vi "I2C Read Byte.vi"(8 "error in (no error)":errorcluster, 10 "Ack? (F:False)":bool, 11 "I2C Task In":T1) -> (0 "error out":errorcluster, 2 "Data Byte":u8 format="%x", 3 "I2C Task Out":T1)   [LabVIEW 2017, in "I2C.lvlib"]
doc: "Reads a single byte from a slave device on the I2C port."
uses:
  <vilib>/robotics/Protocols/I2C/DAQmx/I2C.lvlib
  <vilib>/robotics/Protocols/I2C/DAQmx/Private/I2C Tasks.ctl
  <vilib>/DAQmx/read.llb/DAQmx Read (Digital Bool 1Line 1Point).vi
  <vilib>/DAQmx/miscellaneous.llb/DAQmx Fill In Error Info.vi
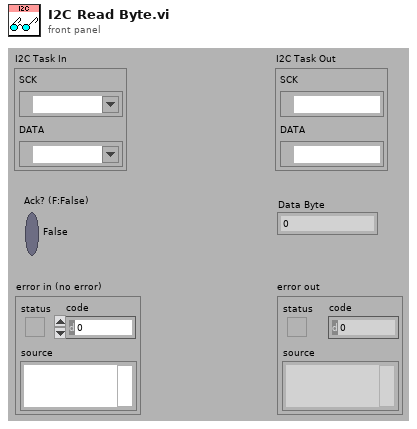
[diagram p1: front panel]
types:
  T1 = typedef "I2C.lvlib/I2C Tasks.ctl" = cluster{"SCK":refnum<k21>, "DATA":refnum<k21>}
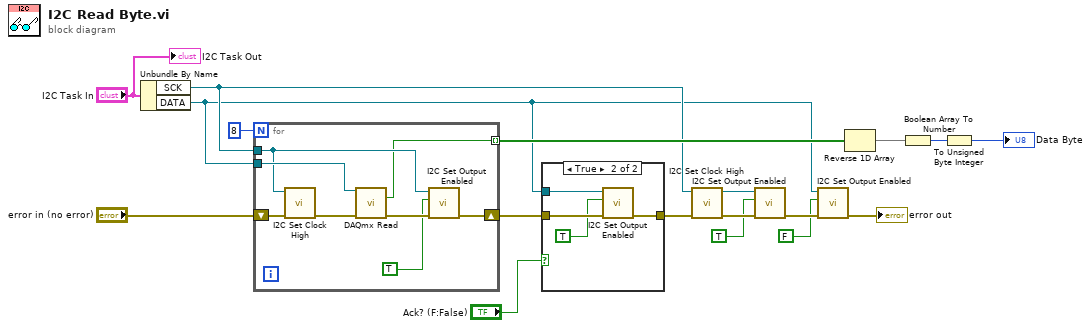
[diagram p0: block diagram]
diagram:
  n1 = Unbundle By Name("I2C Task In") -> ("SCK"=w9:refnum<k21>, "DATA"=w5:refnum<k21>)
  n2 = for {
    N: 8 -> [_]
    shift-right: [w19] -> w11
    shift-left: "error in (no error)" -> [w26]
    tunnel: [w20] -> w14 mode=indexing
    tunnel: w9 -> [w23]
    tunnel: w5 -> [w25]
    n3 = call <vilib>:"I2C Set Clock High.vi"("error in (no error)"=w26, "Task In"=w23) -> ("error out"=w24:errorcluster)  [unwired: 8 in, 1 out]
    n4 = call-poly <vilib>:"DAQmx Read.vi"("task/channels in"=w25, "error in"=w24) -> ("data"=w20:bool, "error out"=w22:errorcluster)  [unwired: 11 in, 1 out]
    n5 = call <vilib>:"I2C Set Output Enabled.vi"("error in (no error)"=w22, "Output Enabled (T:Enable)"=TRUE, "Task In"=w23) -> ("error out"=w19:errorcluster)  [unwired: 7 in, 1 out]
  }
  n6 = case shown="True" "Ack? (F:False)" {
    tunnel: w5 -> [_ w31]
    tunnel: w11 -> [w27 w30]
    tunnel: [w27 w28] -> w10
    frame False {
    }
    frame True {
      n7 = call <vilib>:"I2C Set Output Enabled.vi"("error in (no error)"=w30, "Output Enabled (T:Enable)"=TRUE ("DO.Tristate"), "Task In"=w31) -> ("error out"=w28:errorcluster)  [unwired: 7 in, 1 out]
    }
  }
  n8 = call <vilib>:"I2C Set Clock High.vi"("error in (no error)"=w10, "Task In"=w9) -> ("error out"=w7:errorcluster, "Task Out"=w8:refnum<k21>)  [unwired: 8 in]
  n9 = call <vilib>:"I2C Set Output Enabled.vi"("error in (no error)"=w7, "Output Enabled (T:Enable)"=TRUE ("DO.Tristate"), "Task In"=w8) -> ("error out"=w4:errorcluster)  [unwired: 7 in, 1 out]
  n10 = call <vilib>:"I2C Set Output Enabled.vi"("error in (no error)"=w4, "Output Enabled (T:Enable)"=FALSE ("DO.Tristate"), "Task In"=w5) -> ("error out"=→"error out":errorcluster)  [unwired: 7 in, 1 out]
  n11 = Reverse 1D Array(array=w14) -> (reversed array=w16:bool[])
  n12 = Boolean Array To Number(Boolean array=w16) -> (number=w15:u32)
  n13 = To Unsigned Byte Integer(number=w15) -> (unsigned 8bit integer=→"Data Byte":u8)
  "I2C Task Out" <- "I2C Task In"
